vi "AuMT8852B EDR Fail Register Enable.vi"(5 "Flags (all disabled)":T1 {"Max Input Power" items=["Max input power disabled", "Max input power enabled"]; "BER Floor Sensitivity" items=["BER floor sensitivity disabled", "BER floor sensitivity enabled"]; "Sensitivity" items=["Sensitivity disabled", "Sensitivity enabled"]; "Differential Phase Encoding" items=["Differential phase disabled", "Differential phase enabled"]; "Carrier frequency & Mod" items=["Carrier frequency & mod disabled", "Carrier frequency & mod enabled"]; "Relative Transmit Power" items=["Relative transmit power disabled", "Relative transmit power enabled"]}, 7 "Set/Get (Set)":enum16{"Set", "Get"}(ring), 8 "error in (no error)":errorcluster, 10 "Value (-1)":i32=-1, 11 "VISA session":refnum<visa-resource-name>) -> (0 "error out":errorcluster, 2 "error code":i32, 3 "VISA session out":refnum<visa-resource-name>, 4 "Flags out":T1 {"Max Input Power" items=["Max input power disabled", "Max input power enabled"]; "BER Floor Sensitivity" items=["BER floor sensitivity disabled", "BER floor sensitivity enabled"]; "Sensitivity" items=["Sensitivity disabled", "Sensitivity enabled"]; "Differential Phase Encoding" items=["Differential phase disabled", "Differential phase enabled"]; "Carrier frequency & Mod" items=["Carrier frequency & mod disabled", "Carrier frequency & mod enabled"]; "Relative Transmit Power" items=["Relative transmit power disabled", "Relative transmit power enabled"]}, 6 "Value out":i32)   [LabVIEW 2017]
doc: "Anritsu MT8852B Bluetooth Tester\n\nIndicates which bits of the EDR Equipment Test Fail Register will cause a Service Request (SRQ). The value can be written as an integer (0-255), or as a cluster of flags.\n\nBit 5 (most significant bit) - Maximum input power test.\nBit 4 - BER floor sensitivity test.\nBit 3 - Sensitivity test.\nBit 2 - Differential phase encoding test.\nBit 1 - Carrier stability and modulation accuracy test.\nBit 0 (least significant bit) - Relative transmit power test.\n\nINPUTS\nSet/Get - whether the values are being written to or read from the instrument.\nFlags - individual test bit values to assign to the register.\nValue - integer value (0-255) to be written to the register. Leave this input unwired if you are using the Flags input.\n\nOUTPUTS\nFlags out - status of each test bit in the register.\nValue out - integer value (0-255) of the register."
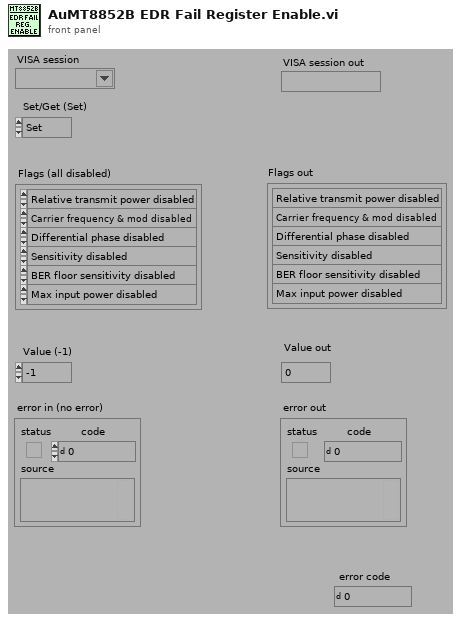
[diagram p1: front panel]
types:
  T1 = cluster{"Relative Transmit Power":u16, "Carrier frequency & Mod":u16, "Differential Phase Encoding":u16, "Sensitivity":u16, "BER Floor Sensitivity":u16, "Max Input Power":u16}
  T2 = enum16{"Simulate", "Range check", "Cache", "Query instrument status"}
  T3 = cluster{"[0]":i16, "[1]":i16, "[2]":i16, "[3]":i16, "[4]":i16, "[5]":i16}
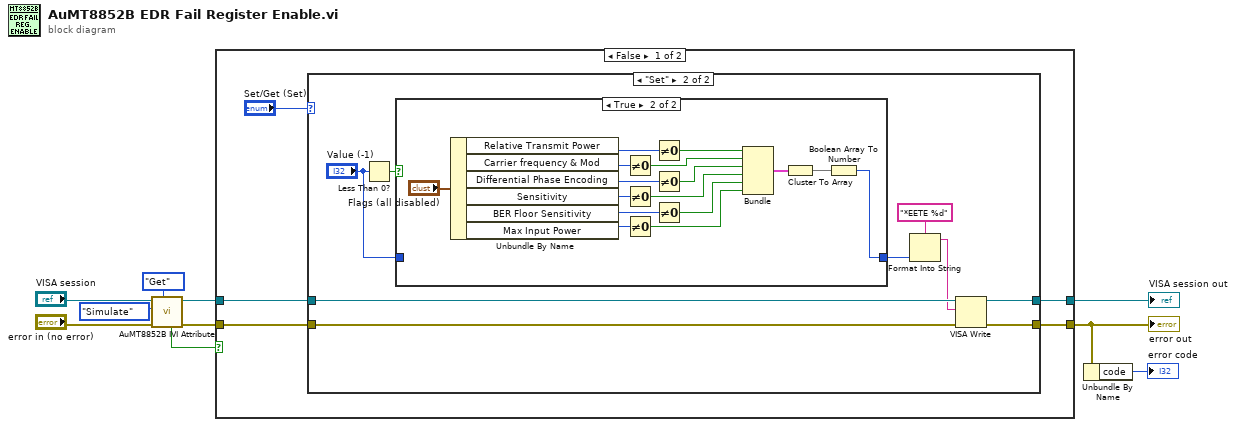
[diagram p0: block diagram]
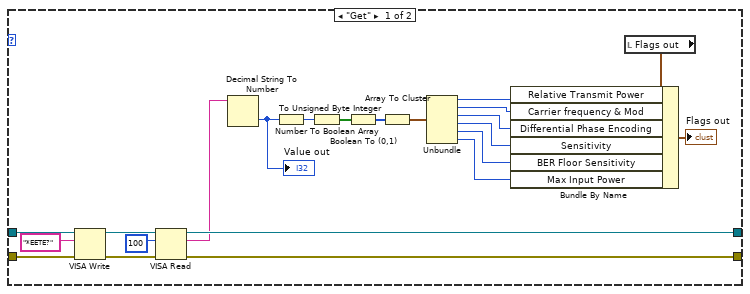
[diagram p2: hidden frame]
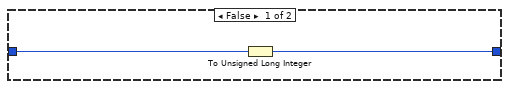
[diagram p3: hidden frame]
diagram:
  n1 = call <instrlib>:"AuMT8852B IVI Attribute.vi"("Set/Get (Set)"=enum16{"Set", "Get"}."Get", "error in (no error)"="error in (no error)", "Flag (Simulate)"=T2."Simulate", "VISA session"="VISA session") -> ("error out"=w6:errorcluster, "VISA session out"=w7:refnum<visa-resource-name>, "Value out"=w3:bool)  [unwired: 5 in]
  n2 = case shown="False" w3 {
    tunnel: [w12 w65] -> w1
    tunnel: [w13 w66] -> w8
    tunnel: w7 -> [w15 w66]
    tunnel: w6 -> [w14 w65]
    frame False {
      n3 = case shown="\"Set\"" "Set/Get (Set)" {
        tunnel: w15 -> [w37 w46]
        tunnel: w14 -> [w36 w45]
        tunnel: [w32 w42] -> w13
        tunnel: [w31 w41] -> w12
        frame "Get" {
          n4 = VISA Write(VISA resource name=w37, write buffer="*EETE?" ("write buffer (\"\")"), error in (no error)=w36) -> (VISA resource name out=w34:refnum<visa-resource-name>, error out=w33:errorcluster)  [unwired: 1 out]
          n5 = VISA Read(VISA resource name=w34, byte count=u32 100 ("byte count (0)"), error in (no error)=w33) -> (VISA resource name out=w32:refnum<visa-resource-name>, read buffer=w29:string, error out=w31:errorcluster)  [unwired: 1 out]
          n6 = Decimal String To Number(string=w29) -> (number=w25:i32)  [unwired: 2 in, 1 out]
          "Value out" <- w25
          n7 = To Unsigned Byte Integer(number=w25) -> (unsigned 8bit integer=w26:u8)
          n8 = Number To Boolean Array(number=w26) -> (Boolean array=w27:bool[])
          n9 = Boolean To (0,1)(Boolean=w27) -> (0, 1=w28:i16[])
          n10 = Array To Cluster(array=w28) -> (cluster=w22:T3)
          n11 = Unbundle(w22) -> ("[0]"=w21:i16, "[1]"=w20:i16, "[2]"=w19:i16, "[3]"=w18:i16, "[4]"=w17:i16, "[5]"=w16:i16)
          n12 = local read "Flags out"() -> (w24:T1)
          n13 = Bundle By Name(cluster=w24, "Relative Transmit Power"=w21, "Carrier frequency & Mod"=w20, "Differential Phase Encoding"=w19, "Sensitivity"=w18, "BER Floor Sensitivity"=w17, "Max Input Power"=w16) -> (→"Flags out":T1)
        }
        frame "Set" {
          n14 = Less Than 0?(x="Value (-1)") -> (x < 0?=w39:bool)
          n15 = case shown="True" w39 {
            tunnel: [w47 w64] -> w43
            tunnel: "Value (-1)" -> [w48 _]
            frame False {
              n16 = To Unsigned Long Integer(number=w48) -> (unsigned 32bit integer=w47:u32)
            }
            frame True {
              n17 = Unbundle By Name("Flags (all disabled)") -> ("Relative Transmit Power"=w57:u16, "Carrier frequency & Mod"=w58:u16, "Differential Phase Encoding"=w59:u16, "Sensitivity"=w60:u16, "BER Floor Sensitivity"=w61:u16, "Max Input Power"=w62:u16)
              n18 = Not Equal To 0?(x=w58) -> (x != 0?=w55:bool)
              n19 = Not Equal To 0?(x=w60) -> (x != 0?=w51:bool)
              n20 = Not Equal To 0?(x=w62) -> (x != 0?=w52:bool)
              n21 = Not Equal To 0?(x=w57) -> (x != 0?=w56:bool)
              n22 = Not Equal To 0?(x=w59) -> (x != 0?=w54:bool)
              n23 = Not Equal To 0?(x=w61) -> (x != 0?=w53:bool)
              n24 = Bundle(w56, w55, w54, w51, w53, w52) -> (w50:cluster{bool, bool, bool, bool, bool, bool})  [unwired: 1 in]
              n25 = Cluster To Array(cluster=w50) -> (array=w49:bool[])
              n26 = Boolean Array To Number(Boolean array=w49) -> (number=w64:u32)
            }
          }
          n27 = Format Into String(format string="*EETE %d" ("Format String"), w43) -> (resulting string=w40:string)  [unwired: 2 in, 1 out]
          n28 = VISA Write(VISA resource name=w46, write buffer=w40, error in (no error)=w45) -> (VISA resource name out=w42:refnum<visa-resource-name>, error out=w41:errorcluster)  [unwired: 1 out]
        }
      }
    }
    frame True {
    }
  }
  "error out" <- w1
  "VISA session out" <- w8
  n29 = Unbundle By Name(w1) -> ("code"=→"error code":i32)
